vi "File List Get Current File.vi"(11 "File List in":refnum<class "File List.lvclass">) -> (1 "Current file index out":i32, 2 "Current file out":path, 3 "File List out":refnum<class "File List.lvclass">)   [LabVIEW 2014, in "COSYLib.lvlib" / "File List.lvclass"]
doc: "Returns the current file (if any).\nNote that \"File Index\" is -1 if the file list is empty."
uses:
  File List.lvclass
  File List.lvclass/File List.ctl
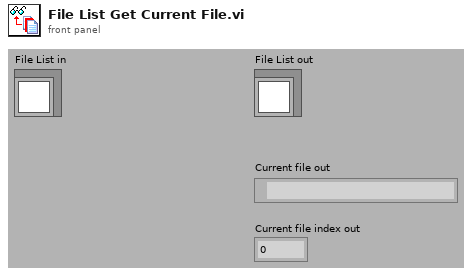
[diagram p1: front panel]
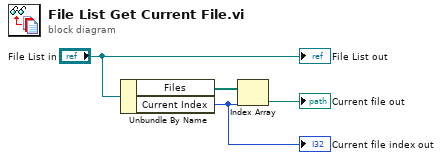
[diagram p0: block diagram]
diagram:
  n1 = Unbundle By Name("File List in") -> ("Files"=w4:path[], "Current Index"=w1:i32)
  "Current file index out" <- w1
  n2 = Index Array(array=w4, index=w1) -> (element=→"Current file out":path)
  "File List out" <- "File List in"
